vi "start.vi"(8 "error in (no error)":errorcluster, 11 "ICCameraAcquisitor in":refnum<class "ICCameraAcquisitor.lvclass">) -> (0 "error out":errorcluster, 3 "ICCameraAcquisitor out":refnum<class "ICCameraAcquisitor.lvclass">)   [LabVIEW 2009, in "Hardware.lvlib" / "Channels.lvlib" / "ICCameraAcquisitor.lvclass"]
uses:
  ICCameraAcquisitor.lvclass
  ICCameraAcquisitor.lvclass/ICCameraAcquisitor.ctl
panel:
  out "CurrentIndex":i32
  out "ImageRingBufferSize":i32
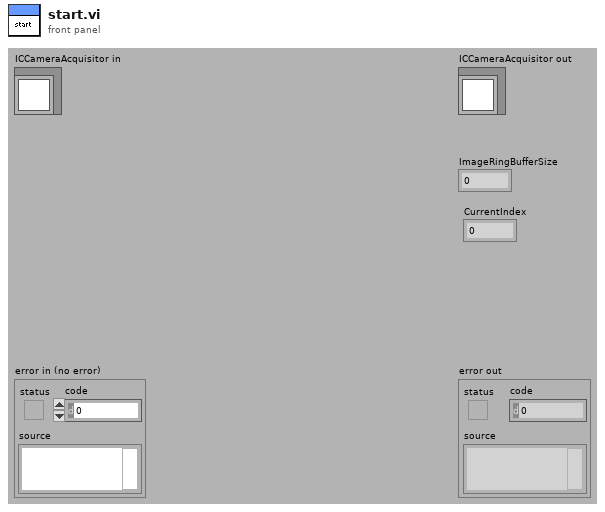
[diagram p1: front panel]
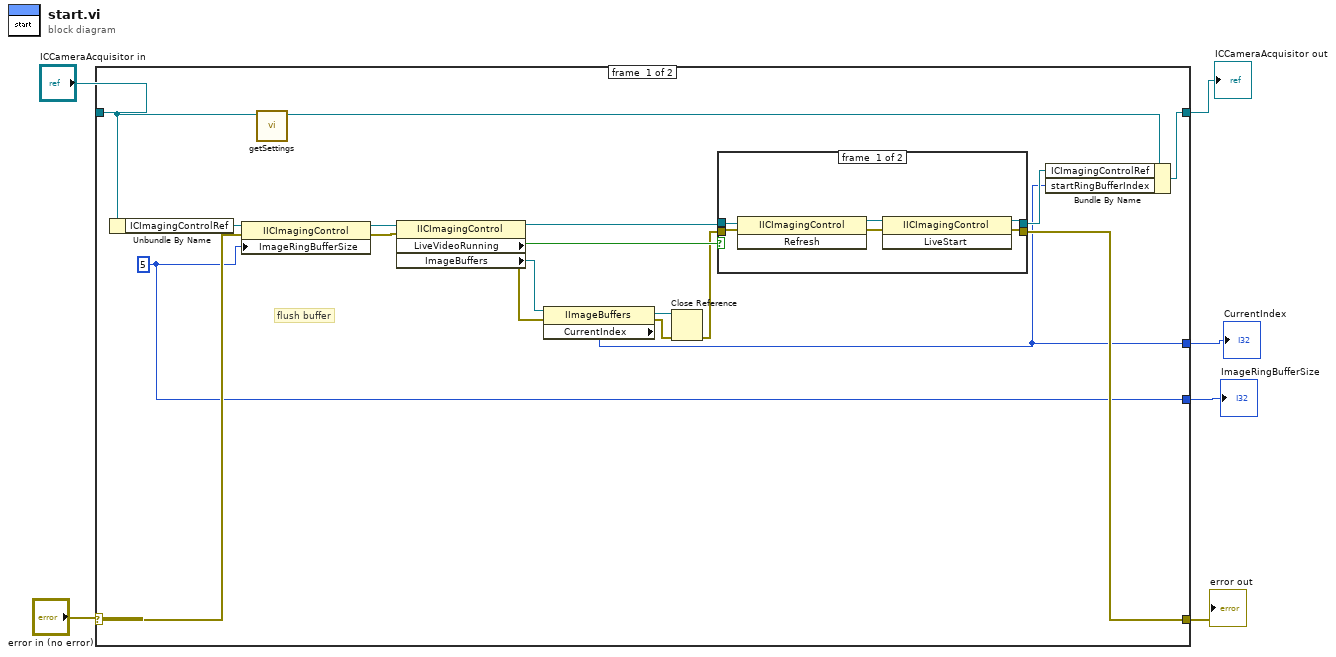
[diagram p0: block diagram]
diagram:
  n1 = case shown="No Error" "error in (no error)" {
    selector: "error in (no error)" -> [w14 w33]
    tunnel: [w16 w33] -> w5
    tunnel: "ICCameraAcquisitor in" -> [w8 w34]
    tunnel: [w22 w34] -> w3
    tunnel: [w11 _] -> w2
    tunnel: [w12 _] -> w1
    frame #0 {
      w11 = 5
      # "flush buffer"
      n2 = Unbundle By Name(w8) -> ("ICImagingControlRef"=w15:refnum<k7>)
      n3 = property class="IICImagingControl"(reference=w15, error in=w14, "ImageRingBufferSize"=w11) -> (reference out=w9:refnum<k7>, error out=w13:errorcluster)
      n4 = call "getSettings.vi"("ICCameraAcquisitor in"=w8) -> ("ICCameraAcquisitor out"=w7:refnum<class "ICCameraAcquisitor.lvclass">)  [unwired: 9 in, 1 out]
      n5 = property class="IICImagingControl"(reference=w9, error in=w13) -> (reference out=w20:refnum<k7>, error out=w21:errorcluster, "LiveVideoRunning"=w24:bool, "ImageBuffers"=w10:refnum<k7>)
      n6 = property class="IImageBuffers"(reference=w10, error in=w21) -> (reference out=w19:refnum<k7>, error out=w18:errorcluster, "CurrentIndex"=w12:i32)
      n7 = Close Reference(reference=w19, error in (no error)=w18) -> (error out=w17:errorcluster)
      n8 = case shown="False" w24 {
        tunnel: w17 -> [w29 w31]
        tunnel: w20 -> [w30 w32]
        tunnel: [w26 w32] -> w23
        tunnel: [w25 w31] -> w16
        frame #0 {
          n9 = invoke class="IICImagingControl" method="Refresh"(reference=w30, error in=w29) -> (reference out=w28:refnum<k7>, error out=w27:errorcluster)  [unwired: 1 in, 1 out]
          n10 = invoke class="IICImagingControl" method="LiveStart"(reference=w28, error in=w27) -> (reference out=w26:refnum<k7>, error out=w25:errorcluster)  [unwired: 1 in, 1 out]
        }
        frame #1 {
        }
      }
      n11 = Bundle By Name(cluster=w7, "ICImagingControlRef"=w23, "startRingBufferIndex"=w12) -> (w22:refnum<class "ICCameraAcquisitor.lvclass">)
    }
    frame #1 {
    }
  }
  "error out" <- w5
  "ICCameraAcquisitor out" <- w3
  "ImageRingBufferSize" <- w2
  "CurrentIndex" <- w1
